vi "prop_format_main.vi"() -> ()   [LabVIEW 2020, in "3DPC_SurfacePlot.xctl"]
uses:
  <vilib>/Native 3D Graph/xcontrol/3DPC_SurfacePlot.xctl
  <vilib>/Native 3D Graph/typedefs/prop_format.ctl
  <vilib>/Utility/miscctls.llb/LVPointTypeDef.ctl
panel:
  in  "Format Strings":i32(listbox)=12
  in  "done":refnum<user-event>
  in  "quit":refnum<user-event>
  out "error out 3":errorcluster
  out "error out 2":errorcluster
  out "error out":errorcluster
  out "Formatted example":string="5.274"
  in  "Example":string="5.274"
  in  "Format string":string
  out "Format Properties Out":T1
  in  "Format Properties In":T1
  in  "Axis":u16(ring) items=["X", "Y", "Z"]
  # "Preview"
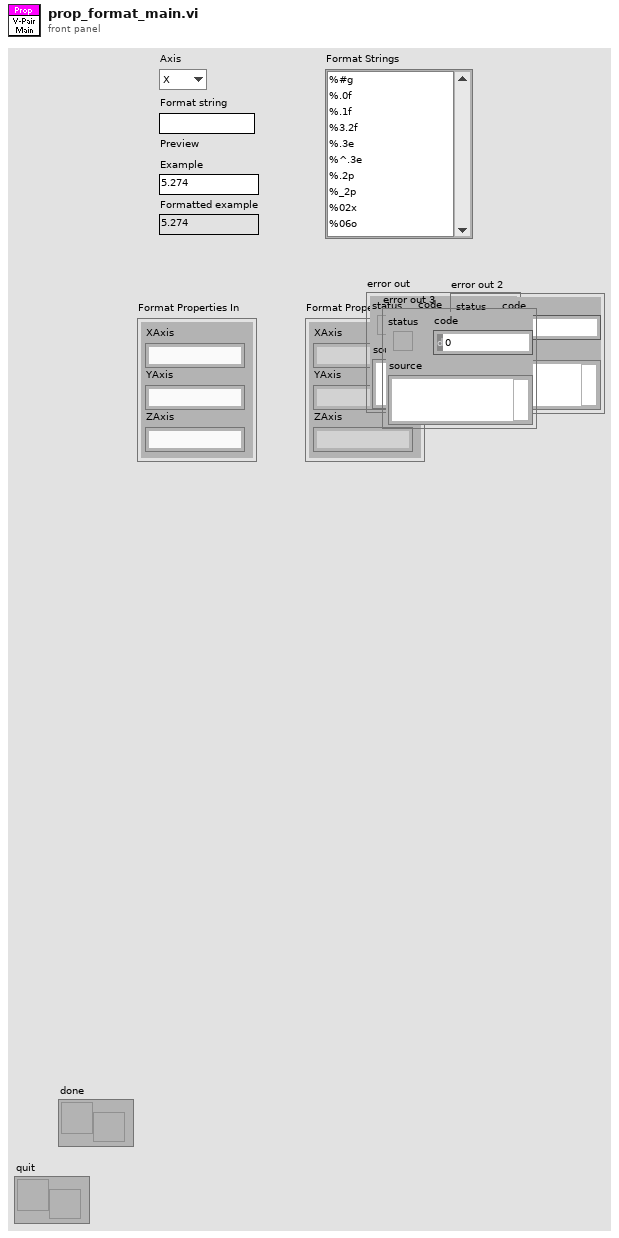
[diagram p1: front panel]
types:
  T1 = typedef "3DPC_SurfacePlot.xctl/prop_format.ctl" = cluster{"XAxis":string, "YAxis":string, "ZAxis":string}
  T2 = typedef "LVPointTypeDef.ctl" = cluster{"Horizontal":i16, "Vertical":i16}
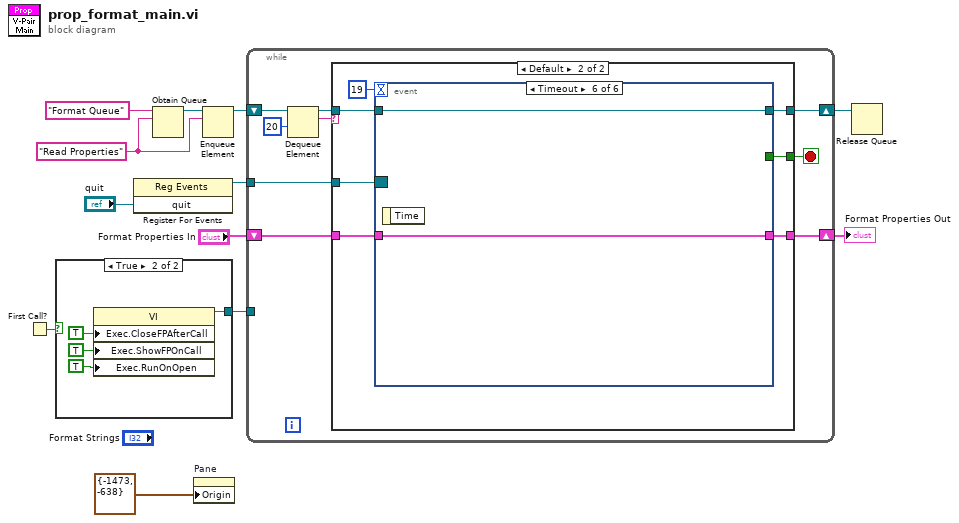
[diagram p0: block diagram]
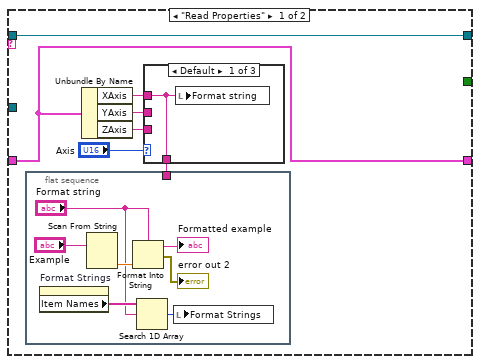
[diagram p3: hidden frame]
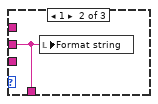
[diagram p4: hidden frame]
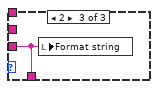
[diagram p5: hidden frame]
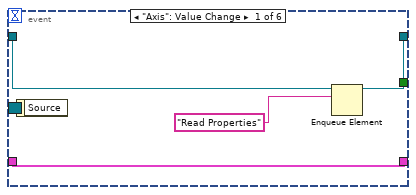
[diagram p6: hidden frame]
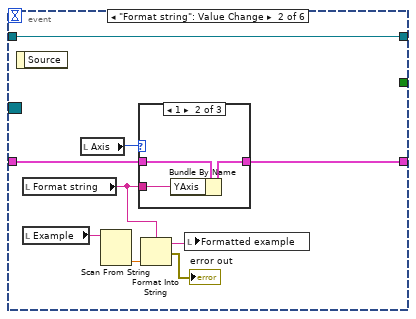
[diagram p7: hidden frame]
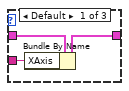
[diagram p8: hidden frame]
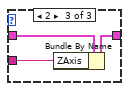
[diagram p9: hidden frame]
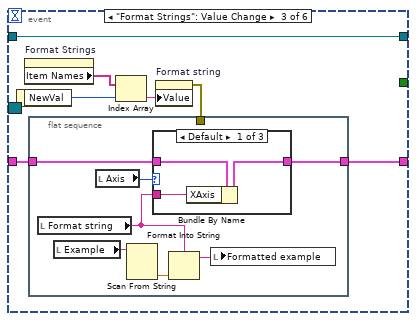
[diagram p10: hidden frame]
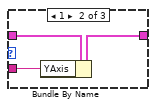
[diagram p11: hidden frame]
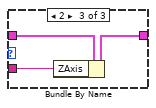
[diagram p12: hidden frame]
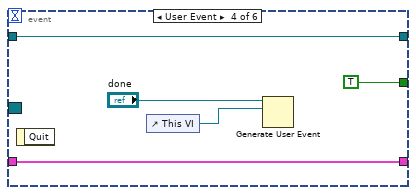
[diagram p13: hidden frame]
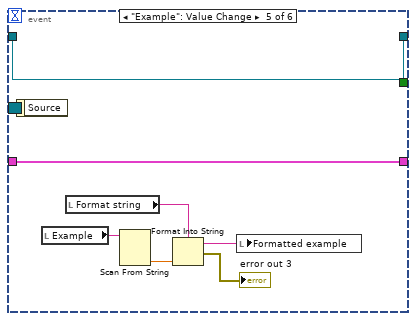
[diagram p14: hidden frame]
diagram:
  w10 = "Read Properties"
  n1 = First Call?() -> (First Call?: T/F=w1:bool)
  n2 = case shown="True" w1 {
    tunnel: [_ w14] -> w7
    frame False {
    }
    frame True {
      n3 = property class="VI"("Exec.CloseFPAfterCall"=TRUE ("Execution:Close After Call"), "Exec.ShowFPOnCall"=TRUE ("Execution:Show Front Panel On Call"), "Exec.RunOnOpen"=TRUE ("Execution:Run When Opened")) -> (reference out=w14:refnum<vi>)  [unwired: 2 in, 1 out]
    }
  }
  n4 = register-events("quit") -> (reference out=w3:refnum<event-registration>)  [unwired: 2 in, 1 out]
  n5 = Obtain Queue(name (unnamed)="Format Queue", element data type=w10) -> (queue out=w11:refnum<queue>)  [unwired: 3 in, 2 out]
  n6 = property on="Pane" class="Pane"("Origin"=T2 {"Horizontal"=-1473, "Vertical"=-638} ("Point")) -> ()  [unwired: 2 in, 2 out]
  n7 = Enqueue Element(queue=w11, element=w10) -> (queue out=w9:refnum<queue>)  [unwired: 1 in, 3 out]
  n8 = while {
    shift-right: [w21] -> w8
    shift-left: w9 -> [w24]
    tunnel: w7 -> [_]
    shift-right: [w19] -> w5
    shift-left: "Format Properties In" -> [w20]
    tunnel: w3 -> [w18]
    stop <- w17 stop-if-true
    n9 = Dequeue Element(queue=w24, timeout in ms (-1)=20) -> (queue out=w22:refnum<queue>, element=w23:string)  [unwired: 1 in, 2 out]
    n10 = case shown="Default" w23 {
      tunnel: w22 -> [w32 w46]
      tunnel: [_ w43] -> w17
      tunnel: [w32 w45] -> w21
      tunnel: w20 -> [w31 w48]
      tunnel: [w31 w47] -> w19
      tunnel: w18 -> [_ w44]
      frame "Read Properties" {
        n11 = flat-sequence {
          tunnel: w27 -> [_]
          frame #0 {
            n12 = property on="Format Strings" class="LstBox (strict)"() -> ("Item Names"=w35:string[])  [unwired: 2 in, 2 out]
            n13 = Scan From String(input string="Example") -> (output 1=w36:dbl)  [unwired: 3 in, 4 out]
            n14 = Format Into String(format string="Format string", w36) -> (resulting string=→"Formatted example":string, error out=→"error out 2":errorcluster)  [unwired: 2 in]
            n15 = Search 1D Array(1D array=w35, element="Format string") -> (index of element=w33:i32)  [unwired: 1 out]
            n16 = local write "Format Strings"(w33) -> ()
          }
        }
        n17 = Unbundle By Name(w31) -> ("XAxis"=w30:string, "YAxis"=w29:string, "ZAxis"=w28:string)
        n18 = case shown="Default" "Axis" {
          tunnel: w30 -> [w40 _ _]
          tunnel: w29 -> [_ w41 _]
          tunnel: w28 -> [_ _ w42]
          tunnel: [w40 w41 w42] -> w27
          frame Default {
            n19 = local write "Format string"(w40) -> ()
          }
          frame 1 {
            n20 = local write "Format string"(w41) -> ()
          }
          frame 2 {
            n21 = local write "Format string"(w42) -> ()
          }
        }
      }
      frame Default {
        n22 = event shown="[5] Timeout" {
          selector: w44 -> [_ _ _ _ _ _]
          dyn-events: _ -> [_ _ _ _ _ _]
          timeout: 19 -> [_ _ _ _ _ _]
          tunnel: w48 -> [w53 w61 w75 w95 w101 w108]
          tunnel: [w53 w60 w73 w95 w101 w108] -> w47
          tunnel: w46 -> [w51 w54 w72 w96 w100 w107]
          tunnel: [w50 w54 w72 w96 w100 w107] -> w45
          tunnel: [_ _ _ TRUE _ _] -> w43
          event "Axis": Value Change {
            n23 = event-data() -> ()  [unwired: 2 out]
            n24 = Enqueue Element(queue=w51, element="Read Properties") -> (queue out=w50:refnum<queue>)  [unwired: 1 in, 3 out]
          }
          event "Format string": Value Change {
            n25 = event-data() -> ()  [unwired: 2 out]
            n26 = local read "Format string"() -> (w57:string)
            n27 = local read "Example"() -> (w59:string)
            n28 = local read "Axis"() -> (w62:u16)
            n29 = Scan From String(input string=w59) -> (output 1=w58:dbl)  [unwired: 3 in, 4 out]
            n30 = case shown="1" w62 {
              tunnel: w61 -> [w65 w67 w70]
              tunnel: w57 -> [w64 w66 w69]
              tunnel: [w63 w68 w71] -> w60
              frame Default {
                n31 = Bundle By Name(cluster=w65, "XAxis"=w64) -> (w63:T1)
              }
              frame 1 {
                n32 = Bundle By Name(cluster=w67, "YAxis"=w66) -> (w68:T1)
              }
              frame 2 {
                n33 = Bundle By Name(cluster=w70, "ZAxis"=w69) -> (w71:T1)
              }
            }
            n34 = Format Into String(format string=w57, w58) -> (resulting string=w56:string, error out=→"error out":errorcluster)  [unwired: 2 in]
            n35 = local write "Formatted example"(w56) -> ()
          }
          event "Format Strings": Value Change {
            n36 = event-data() -> ("NewVal"=w77:i32)  [unwired: 1 out]
            n37 = property on="Format Strings" class="LstBox (strict)"() -> ("Item Names"=w78:string[])  [unwired: 2 in, 2 out]
            n38 = flat-sequence {
              tunnel: w75 -> [w82]
              tunnel: w74 -> [_]
              tunnel: [w81] -> w73
              frame #0 {
                n39 = local read "Format string"() -> (w79:string)
                n40 = local read "Example"() -> (w84:string)
                n41 = local read "Axis"() -> (w85:u16)
                n42 = Scan From String(input string=w84) -> (output 1=w80:dbl)  [unwired: 3 in, 4 out]
                n43 = case shown="Default" w85 {
                  tunnel: w82 -> [w88 w90 w93]
                  tunnel: w79 -> [w87 w89 w92]
                  tunnel: [w86 w91 w94] -> w81
                  frame Default {
                    n44 = Bundle By Name(cluster=w88, "XAxis"=w87) -> (w86:T1)
                  }
                  frame 1 {
                    n45 = Bundle By Name(cluster=w90, "YAxis"=w89) -> (w91:T1)
                  }
                  frame 2 {
                    n46 = Bundle By Name(cluster=w93, "ZAxis"=w92) -> (w94:T1)
                  }
                }
                n47 = Format Into String(format string=w79, w80) -> (resulting string=w83:string)  [unwired: 2 in, 1 out]
                n48 = local write "Formatted example"(w83) -> ()
              }
            }
            n49 = Index Array(array=w78, index=w77) -> (element=w76:string)
            n50 = property on="Format string" class="Str"("Value"=w76) -> (error out=w74:errorcluster)  [unwired: 2 in, 1 out]
          }
          event User Event {
            n51 = event-data() -> ()  [unwired: 2 out]
            n52 = control-ref of="This VI"() -> (w97:refnum<vi>)
            n53 = Generate User Event(user event="done", event data cluster=w97) -> ()  [unwired: 2 in, 2 out]
          }
          event "Example": Value Change {
            n54 = event-data() -> ()  [unwired: 2 out]
            n55 = local read "Example"() -> (w106:string)
            n56 = local read "Format string"() -> (w104:string)
            n57 = Scan From String(input string=w106) -> (output 1=w105:dbl)  [unwired: 3 in, 4 out]
            n58 = Format Into String(format string=w104, w105) -> (resulting string=w103:string, error out=→"error out 3":errorcluster)  [unwired: 2 in]
            n59 = local write "Formatted example"(w103) -> ()
          }
          event Timeout {
            n60 = event-data() -> ()  [unwired: 2 out]
          }
        }
      }
    }
  }
  "Format Properties Out" <- w5
  n61 = Release Queue(queue=w8) -> ()  [unwired: 1 in, 4 out]
